vi "test_CRC-U32 - Check Protection with corrupt data.vi"(8 "error in (no error)":errorcluster) -> (0 "error out":errorcluster)   [LabVIEW 2023, in "Instrument Addon Protections Unit Tests.lvclass"]
uses:
  Instrument Addon Protections Unit Tests.lvclass
  <vilib>/addons/_JKI Toolkits/VI Tester/TestCase.llb/TestCase.lvclass
  CRC-32/CRC-32.lvclass
panel:
  out "CRC-32 out":refnum<class "CRC-32.lvclass">
  in  "CRC-32 in":refnum<class "CRC-32.lvclass">
  out "TestCase out":refnum<class "Instrument Addon Protections Unit Tests.lvclass">
  in  "TestCase in":refnum<class "Instrument Addon Protections Unit Tests.lvclass">
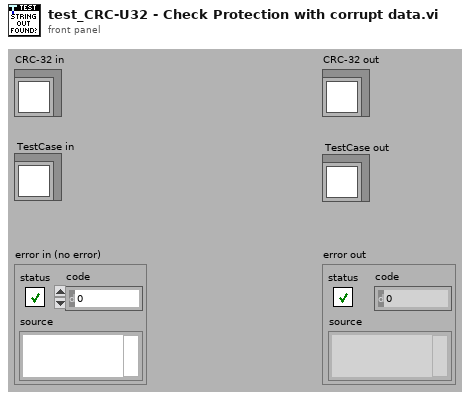
[diagram p1: front panel]
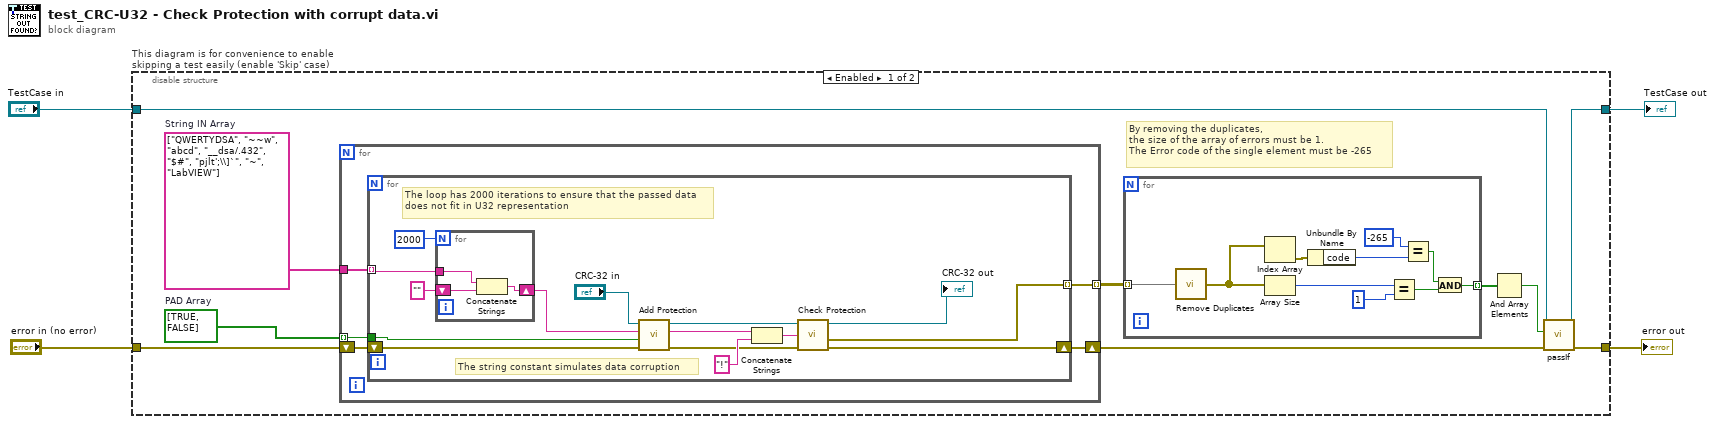
[diagram p0: block diagram]
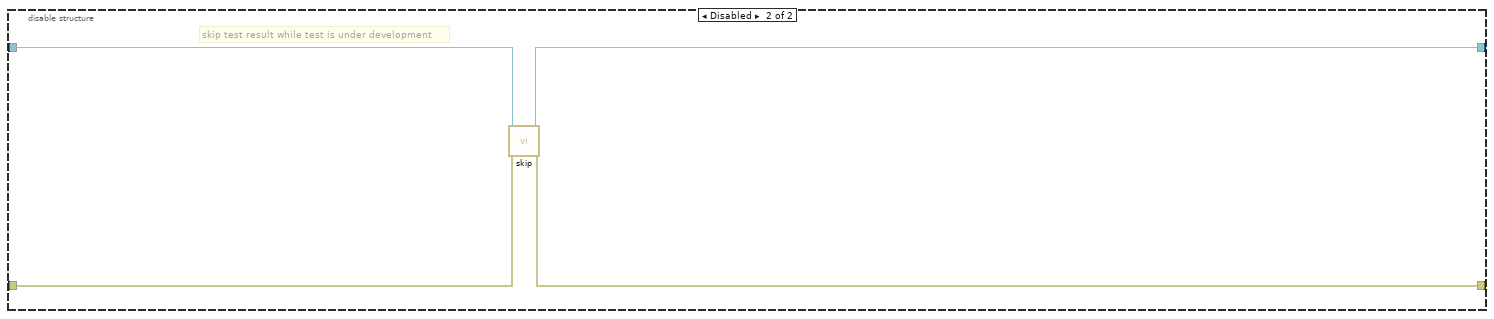
[diagram p2: hidden frame]
diagram:
  n1 = disable-structure "This diagram is for convenience to enable skipping a test easily (enable 'Skip' case)" shown="Enabled" {
    disable-tunnel: "TestCase in" -> [w12 w51]
    disable-tunnel: [w11 w49] -> w1
    disable-tunnel: [w10 w50] -> w3
    disable-tunnel: "error in (no error)" -> [w14 w48]
    frame Enabled {
      w8 = bool[] [TRUE, FALSE]  # PAD Array
      w13 = string[] ["QWERTYDSA", "~~w", "abcd", "__dsa/.432", "$#", "pjlt';\\]`", "~", "LabVIEW"]  # String IN Array
      # "By removing the duplicates, \nthe size of the array of errors must be 1. \nThe Error code of the single element must be -265"
      n2 = for {
        tunnel: w13 -> [w28]
        tunnel: [w26] -> w5 mode=indexing
        shift-right: [w27] -> w9
        shift-left: w14 -> [w29]
        tunnel: w8 -> [w25] mode=indexing
        n3 = for {
          tunnel: w28 -> [w42] mode=indexing
          shift-right: [w37] -> w27
          shift-left: w29 -> [w36]
          tunnel: [w38] -> w26 mode=indexing
          tunnel: w25 -> [w30]
          # "The string constant simulates data corruption"
          # "The loop has 2000 iterations to ensure that the passed data\ndoes not fit in U32 representation"
          n4 = for {
            N: 2000 -> [_]
            shift-right: [w47] -> w35
            shift-left: "" -> [w46]
            tunnel: w42 -> [w45]
            n5 = Concatenate Strings(w45, w46) -> (w47:string)
          }
          n6 = call-dynamic "Add Protection.vi"("error in (no error)"=w36, "Pad"=w30, "String in"=w35, "CRC-32 in"="CRC-32 in") -> ("error out"=w33:errorcluster, "String out"=w32:string, "CRC-32 out"=w31:refnum<class "CRC-32.lvclass">)  [unwired: 5 in]
          n7 = Concatenate Strings(w32, "!" ("string")) -> (w40:string)
          n8 = call-dynamic "Check Protection.vi"("error in (no error)"=w33, "String in"=w40, "CRC-32 in"=w31) -> ("error out"=w37:errorcluster, "Protection Error"=w38:errorcluster, "CRC-32 out"=→"CRC-32 out":refnum<class "CRC-32.lvclass">)  [unwired: 5 in, 1 out]
        }
      }
      n9 = for {
        tunnel: w5 -> [w24] mode=indexing
        tunnel: [w19] -> w6 mode=indexing
        n10 = call "Remove Duplicates.vi"("Array In"=w24) -> ("Array Out"=w20:errorcluster[])
        n11 = Index Array(array=w20) -> (element=w16:errorcluster)  [unwired: 1 in]
        n12 = Array Size(array=w20) -> (size(s)=w15:i32)
        n13 = Unbundle By Name(w16) -> ("code"=w17:i32)
        n14 = Equal?(x=w15, y=1) -> (x = y?=w21:bool)
        n15 = Equal?(x=-265, y=w17) -> (x = y?=w22:bool)
        n16 = And(x=w22, y=w21) -> (x .and. y?=w19:bool)
      }
      n17 = And Array Elements(Boolean array=w6) -> (logical AND=w7:bool)
      n18 = call-dynamic "passIf.vi"("error in (no error)"=w9, "pass"=w7, "TestCase in"=w12) -> ("error out"=w10:errorcluster, "TestCase out"=w11:refnum<class "Instrument Addon Protections Unit Tests.lvclass">)  [unwired: 7 in]
    }
    frame Disabled {
      # "skip test result while test is under development"
      n19 = call <vilib>:"skip.vi"("error in (no error)"=w48, "TestCase in"=w51) -> ("error out"=w50:errorcluster, "TestCase out"=w49:refnum<class "Instrument Addon Protections Unit Tests.lvclass">)  [unwired: 8 in]
    }
  }
  "error out" <- w3
  "TestCase out" <- w1
